vi "Configure Charge Measurement (Offset).vi"(6 "Auto Charge Offset (T: Enable)":bool=TRUE, 7 "Enable Charge Offset (F: Disable)":bool, 8 "error in (no error)":errorcluster, 9 "Charge Offset (0)":dbl, 10 "Channel (1: Channel 1)":i32(ring)=1 items=["Channel 1"=1, "Channel 2"=2], 11 "VISA resource name":refnum<visa-resource-name>) -> (0 "error out":errorcluster, 3 "VISA resource name out":refnum<visa-resource-name>)   [LabVIEW 2012, in "Keysight B2980 Series.lvlib"]
doc: "Configures the offset settings for charge measurement function.\n\n<b>Note(s):</b>\n(1) This VI is only applicable for model B2985A and B2987A.\n(2) Charge measurement should be enabled from <b>Configure Measurement Function.vi</b>."
uses:
  Keysight B2980 Series.lvlib
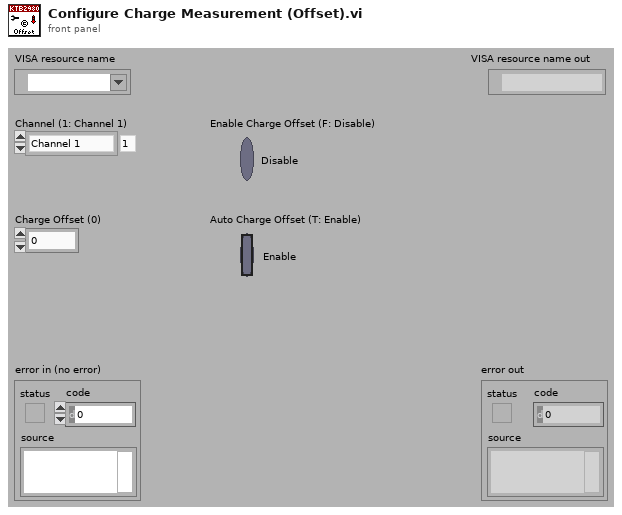
[diagram p1: front panel]
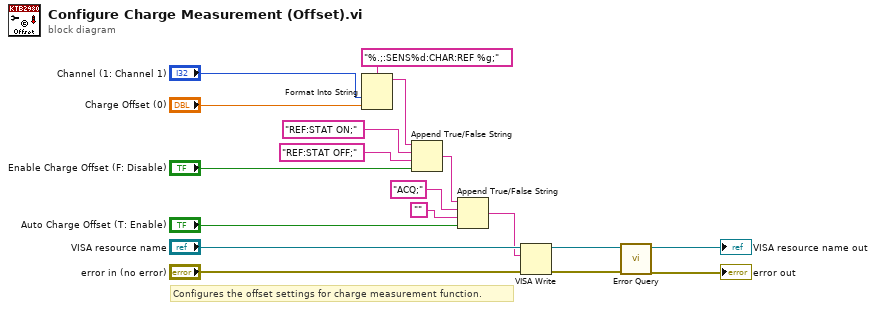
[diagram p0: block diagram]
diagram:
  # "Configures the offset settings for charge measurement function."
  n1 = Format Into String(format string="%.;:SENS%d:CHAR:REF %g;", "Channel (1: Channel 1)", "Charge Offset (0)") -> (resulting string=w7:string)  [unwired: 2 in, 1 out]
  n2 = Append True/False String(1:"Enable Charge Offset (F: Disable)", 2:"REF:STAT OFF;", 3:"REF:STAT ON;", 4:w7) -> (0:w6:string)
  n3 = Append True/False String(1:"Auto Charge Offset (T: Enable)", 2:"", 3:"ACQ;", 4:w6) -> (0:w5:string)
  n4 = VISA Write(VISA resource name="VISA resource name", write buffer=w5, error in (no error)="error in (no error)") -> (VISA resource name out=w16:refnum<visa-resource-name>, error out=w15:errorcluster)  [unwired: 1 out]
  n5 = call "Error Query.vi"("error in (no error)"=w15, "VISA resource name"=w16) -> ("error out"=→"error out":errorcluster, "VISA resource name out"=→"VISA resource name out":refnum<visa-resource-name>)  [unwired: 8 out]
